vi "DAQ_Dig PWM Meas Initialize.vi"(0 "Physical Channel (counter)":tag, 2 "Input Terminal":tag, 7 "Global Channel (counter)":refnum<k21>, 11 "error in":errorcluster) -> (4 "DAQmx Task Out":refnum<k21>, 15 "error out":errorcluster)   [LabVIEW 2021, in "DAQ_Digital PWM Measurement.lvlib"]
doc: "Initialize Counter Input task for digital PWM measurement.\n\nProvide either Physical channel or Global channel for counters to use.\nIf both physical and global channels are provided, Global Channels will take precedence\n\nNote: There cannot be multiple counters in the same task for input operations. Use a separate task for each counter."
uses:
  DAQ_Digital PWM Measurement.lvlib
  <vilib>/DAQmx/create/channels.llb/DAQmx Create Channel (CI-Semi Period).vi
  <resource>/objmgr/daqmx.rc
panel:
  # "Inputs"
  # "Outputs"
  # "Overview:\nThis VI initializes a counter input channel for digital PWM measurement and provides the DAQmx Task Out\n\nHardware Requirement: A compatible PXI, PCIe, USB, cDAQ or Testscale device\n\nSoftware Requirement: NI DAQmx 2022Q4 or later\n\nInstructions:\n1. Enter Input Terminal on which the signal to be measured. Refer Help for more details on the default terminals of each counters. User can configure different PFI lines as well. \n2. Enter counter which should be used for Digital PWM Measurement in Physical Channel (counter) control (Or) Enter Global virtual counters under Global Channel (counter) control to use it instead of initiating a new task. User must configure only one input. If both are provided, Global Channel (counter) will take precedence.\n3. Get the Digital PWM measurement task from DAQmx Task Out which stores the reference to the virtual counter input channel.\n\nNotes: \n1. User can use the DAQmx Task on other VI in this library to configure and initiate digital PWM measurement task.\n2. Multiple counters cannot be initialized in the same task, Use a separate task for each counter.\n3. Global Channel (Counter) input terminal supports only Semi-Period Counter Input global channels from NI MAX. The VI returns error for other invalid global channels.\n4. During Initialize, the counters are reserved with default timebase (default 80MHz timebase for TestScale). For more details to modify the counter timebase, refer the detailed help section."
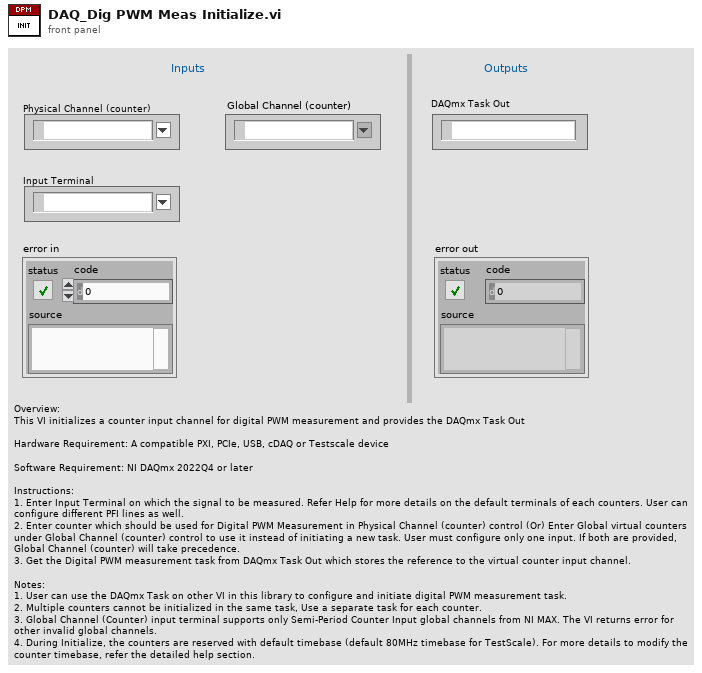
[diagram p1: front panel]
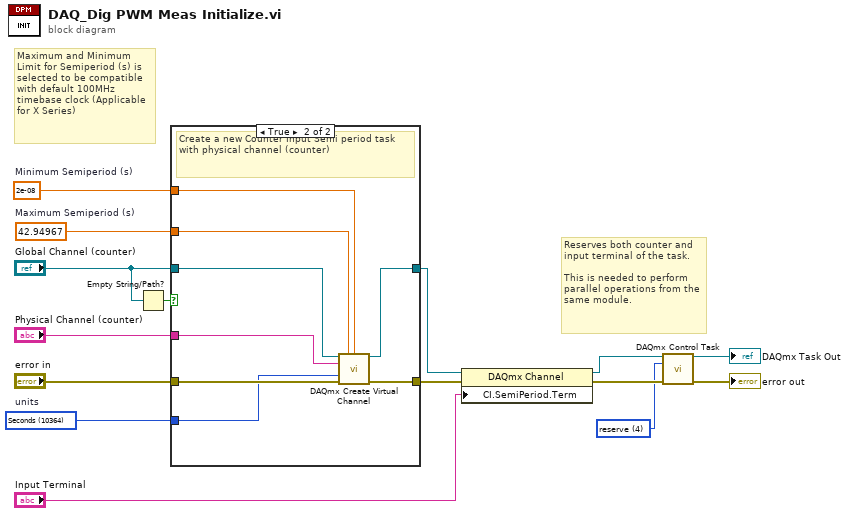
[diagram p0: block diagram]
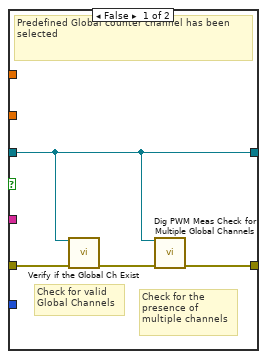
[diagram p2: hidden frame]
diagram:
  w1 = 42.94967  # Maximum Semiperiod (s)
  w2 = 2e-08  # Minimum Semiperiod (s)
  w3 = 10364 items=["Seconds"=10364, "Ticks"=10304, "From Custom Scale"=10065]  # units
  w5 = 4 items=["verify"=2, "reserve"=4, "commit"=3, "unreserve"=5, "abort"=6] ("action")
  # "Maximum and Minimum Limit for Semiperiod (s) is selected to be compatible with default 100MHz timebase clock (Applicable for X Series)"
  # "Reserves both counter and input terminal of the task.\n\nThis is needed to perform parallel operations from the same module."
  n1 = Empty String/Path?(string/path="Global Channel (counter)") -> (empty?=w13:bool)
  n2 = case shown="True" w13 {
    tunnel: "Physical Channel (counter)" -> [_ w24]
    tunnel: "Global Channel (counter)" -> [w16 w27]
    tunnel: [w16 w26] -> w4
    tunnel: "error in" -> [w19 w25]
    tunnel: [w17 w23] -> w11
    tunnel: w3 -> [_ w22]
    tunnel: w2 -> [_ w21]
    tunnel: w1 -> [_ w20]
    frame False {
      # "Check for the\npresence of \nmultiple channels"
      # "Check for valid \nGlobal Channels"
      # "Predefined Global counter channel has been selected"
      n3 = call "Verify if the Global Ch Exist.vi"("Global Channels"=w16, "error in (no error)"=w19) -> ("error out"=w18:errorcluster)  [unwired: 13 in]
      n4 = call "Dig PWM Meas Check for Multiple Global Channels.vi"("Global Channel In"=w16, "error in (no error)"=w18) -> ("error out"=w17:errorcluster)  [unwired: 12 in, 1 out]
    }
    frame True {
      # "Create a new Counter Input Semi period task with physical channel (counter)"
      n5 = call-poly <vilib>:"DAQmx Create Virtual Channel.vi"("task in"=w27, "maximum value"=w20, "minimum value"=w21, "counter"=w24, "units"=w22, "error in"=w25) -> ("task out"=w26:refnum<k21>, "error out"=w23:errorcluster)  [unwired: 8 in]
    }
  }
  n6 = property class="DAQmx Channel"(reference=w4, error in=w11, "CI.SemiPeriod.Term"="Input Terminal") -> (reference out=w7:refnum<k21>, error out=w9:errorcluster)
  n7 = call <vilib>:"DAQmx Control Task.vi"("task/channels in"=w7, "action"=w5, "error in"=w9) -> ("task out"=→"DAQmx Task Out":refnum<k21>, "error out"=→"error out":errorcluster)  [unwired: 11 in]
